vi "KRION6T_termo_main__.vi"() -> ()   [LabVIEW 2015]
doc: "Термометрия КРИОН-6Т"
uses:
  <vilib>/NI/Modbus Library/API/Master/Modbus Master.lvclass
  <vilib>/Utility/error.llb/DialogType.ctl
panel:
  in  "счетчик":u16
  out "Связь с блоком":bool
  in  "Tab Control":enum32{"ИЗМЕРЕНИЯ", "НАСТРОЙКИ"}(tab)
  out "Alarm":bool
  out "разница Т":dbl format="%.2f"
  in  "4_ch_visible":bool=TRUE
  in  "3_ch_visible":bool=TRUE
  out "R2":dbl format="%.2f"
  out "R1":dbl format="%.2f"
  in  "2_ch_visible":bool=TRUE
  in  "1_ch_visible":bool=TRUE
  out "Спаи":dbl format="%.2f"
  out "Cтр.":dbl format="%.2f"
  out "Пер.":dbl format="%.2f"
  out "Сол.":dbl format="%.2f"
  out "R3":dbl format="%.2f"
  out "R4":dbl format="%.2f"
  in  "Т min":dbl=4.0 min=-10.0 max=350.0 step=0.1
  in  "Т max":dbl=350.0 min=2.0 max=500.0 step=0.1
  in  "Autoscale":bool=TRUE
  out "сек.":string="0"
  out "часы":string="0"
  in  "Добавить время":dbl(ring)=300.0 items=["10 сек."=10.0, "1 мин."=60.0, "5 мин."=300.0, "20 мин."=1200.0]
  out "мин.":string="1"
  in  "xScale +":bool
  in  "xScale -":bool
  in  "Сохранение в файл":bool
  in  "Buf_size":u16=10 min=1 max=128
  in  "SPS":T1(ring)=enum."5 SPS"
  out "Путь к файлу с коэффициентами":path
  in  "Пароль":string
  in  "настр. коэфф.":bool caption="Disconn"
  in  "К спаи":T2 {"R0" format="%#_16g"; "k7" format="%#_16g"; "k6" format="%#_16g"; "k5" format="%#_16g"; "k4" format="%#_16g"; "k3" format="%#_16g"; "k2" format="%#_16g"; "k1" format="%#_16g"}
  in  "load_coeff.":bool caption="Disconn"
  in  "save_coeff.":bool caption="Disconn"
  in  "stop":bool
  in  "К стр.":T2 {"R0" format="%#_16g"; "k7" format="%#_16g"; "k6" format="%#_16g"; "k5" format="%#_16g"; "k4" format="%#_16g"; "k3" format="%#_16g"; "k2" format="%#_16g"; "k1" format="%#_16g"}
  in  "GraphLookB":bool
  in  "IP":string
  in  "Порт":u16
  in  "К пер.":T2 {"R0" format="%#_16g"; "k7" format="%#_16g"; "k6" format="%#_16g"; "k5" format="%#_16g"; "k4" format="%#_16g"; "k3" format="%#_16g"; "k2" format="%#_16g"; "k1" format="%#_16g"}
  in  "К сол.":T2 {"R0" format="%#_16g"; "k7" format="%#_16g"; "k6" format="%#_16g"; "k5" format="%#_16g"; "k4" format="%#_16g"; "k3" format="%#_16g"; "k2" format="%#_16g"; "k1" format="%#_16g"}
  out "Path":string
  in  "интервал сохр.":u16=10 min=1 max=3600 step=1
  out "Сутки":string
  in  "Запись в файл":bool
  out "File header exist?":bool caption="Disconn"
  in  "ADC_dyn_range":T3(ring)=enum."± 0.625 В"
  out "refnum out":refnum<file>
  out "Graphs T":dynamicdata(graph) caption="ИЗМЕРЕНИЯ ТЕМПЕРАТУРЫ, К"
  out "Связь":refnum<class "Modbus Master.lvclass">
  in  "Buf_size":u8=1 min=1 max=128
  in  "SPS":T1(ring)
  out "Расположение файла":path
  # "Т [K]"
  # "R [Ом]"
  # "сол./спаи dT ="
  # "Больше 40 К ?"
  # ":"
  # ":"
  # "Шкала Т"
  # "id 103"
  # "Скорость измерений"
  # "Размер буфера усредн."
  # "SPS = Samples Per Second"
  # "сек."
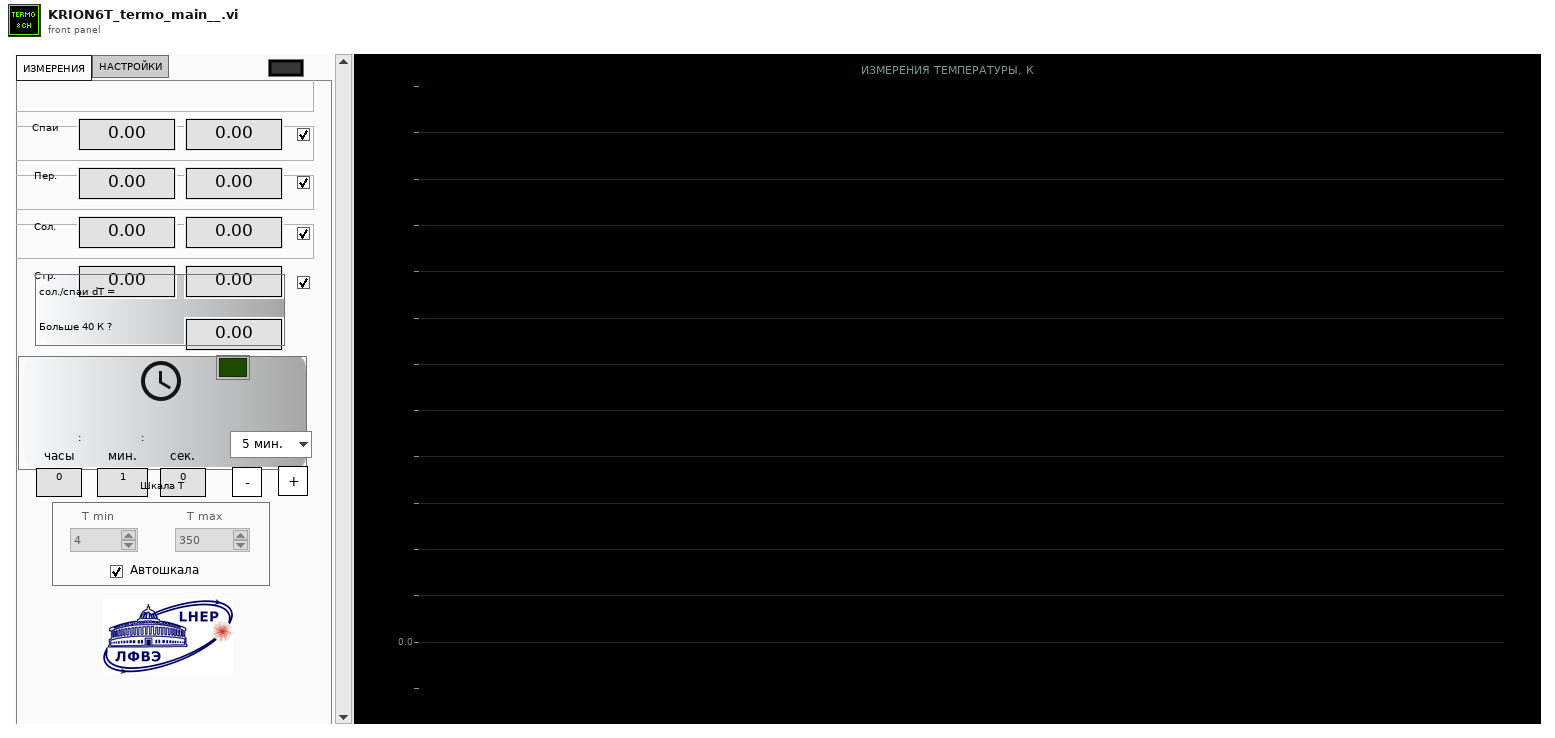
[diagram p1: front panel]
types:
  T1 = enum16{"2,5 SPS", "5 SPS", "10 SPS", "25 SPS", "50 SPS", "100 SPS", "500 SPS", "1 kSPS"}
  T2 = cluster{"k1":ext, "k2":ext, "k3":ext, "k4":ext, "k5":ext, "k6":ext, "k7":ext, "R0":ext}
  T3 = enum16{"± 5 В", "± 2.5 В", "± 1.25 В", "± 0.625 В", "± 312.5 мВ", "± 156.25 мВ", "± 78.125 мВ"}
  T4 = typedef "DialogType.ctl" = u16
  T5 = enum8{"Enabled", "Disabled", "Disabled and Grayed Out"}
  T6 = typedef "LVDateTimeRec.ctl" = cluster{"fractional second":dbl, "second":i32, "minute":i32, "hour":i32, "day of month":i32, "month":i32, "year":i32, "day of week":i32, "day of year":i32, "DST":i32}
  T7 = enum16{"open", "replace", "create", "open or create", "replace or create", "replace or create with confirmation"}
  T8 = cluster{"k1":ext, "k2":ext, "k3":ext, "k4":ext, "k5":ext, "k6":ext, "k7":ext, "R":ext}
  T9 = cluster{"Cтр.":dbl, "Спаи":dbl, "Пер.":dbl, "Сол.":dbl}
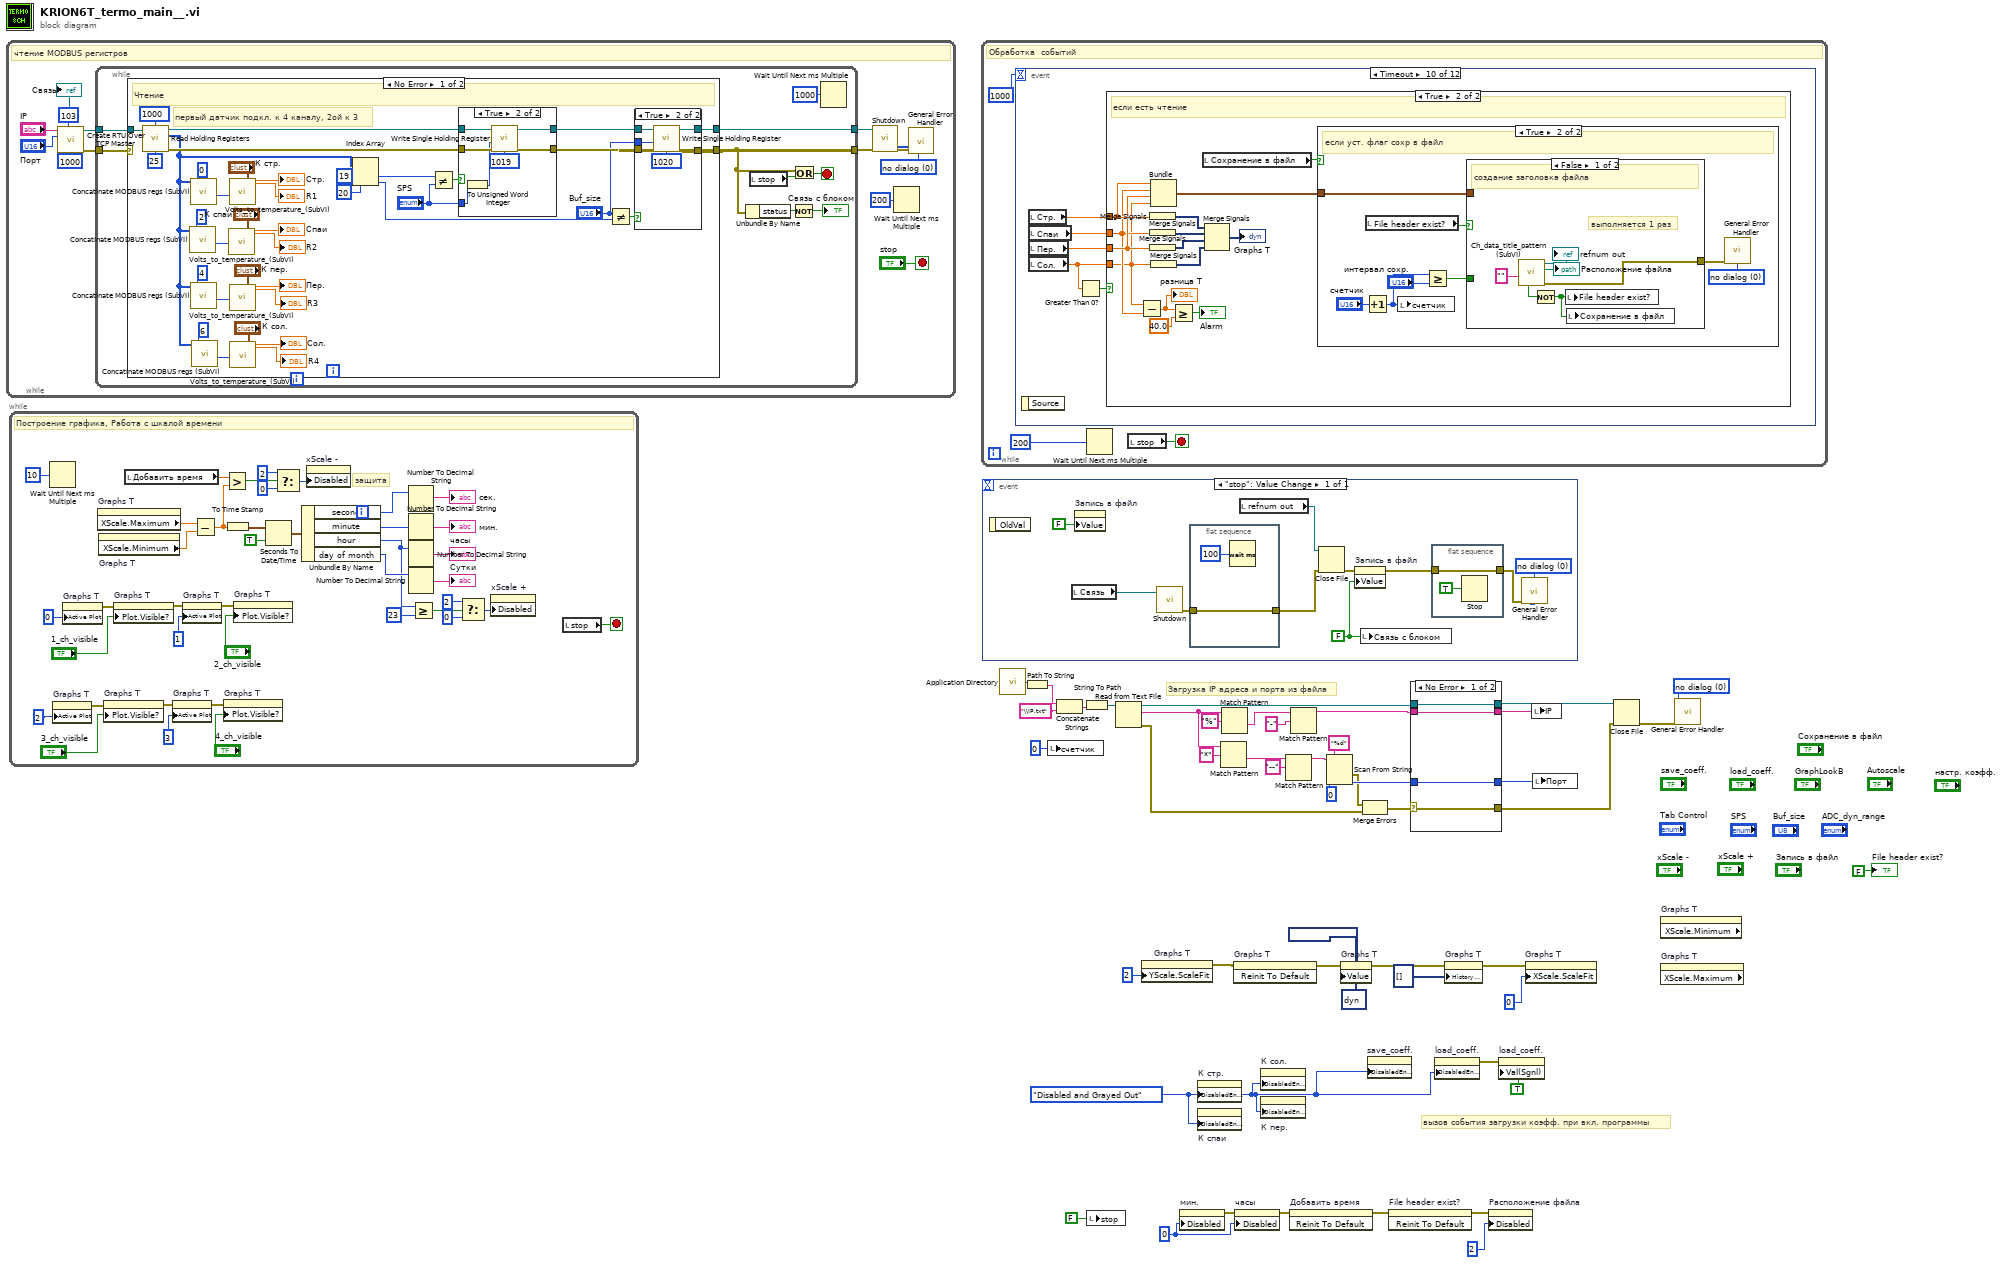
[diagram p0: block diagram]
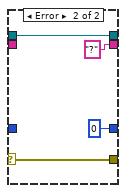
[diagram p2: hidden frame]
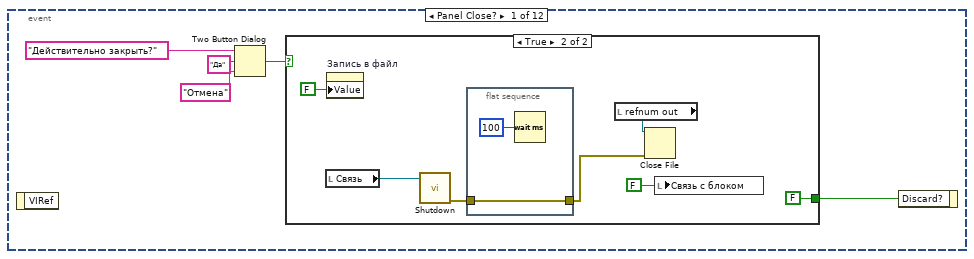
[diagram p3: hidden frame]
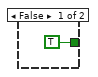
[diagram p4: hidden frame]
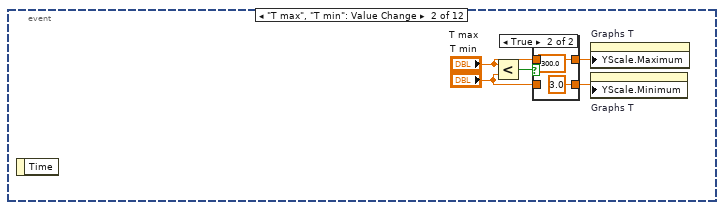
[diagram p5: hidden frame]
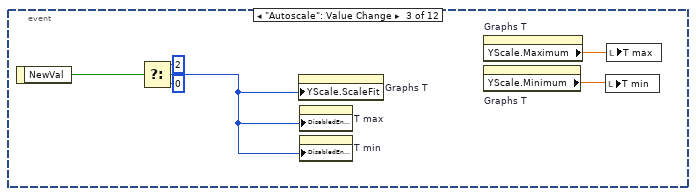
[diagram p7: hidden frame]
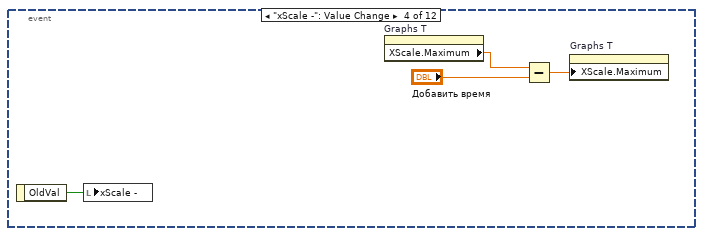
[diagram p8: hidden frame]
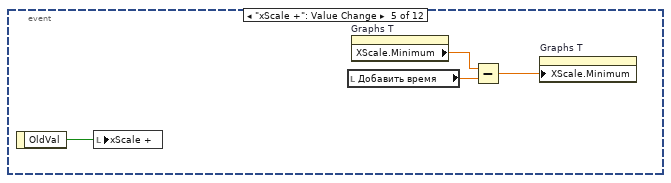
[diagram p9: hidden frame]
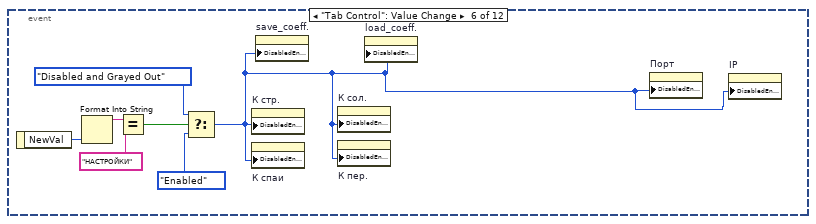
[diagram p10: hidden frame]
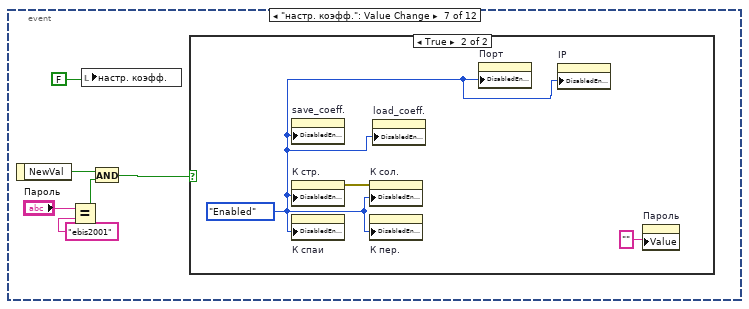
[diagram p11: hidden frame]
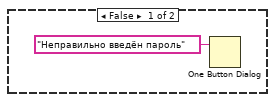
[diagram p12: hidden frame]
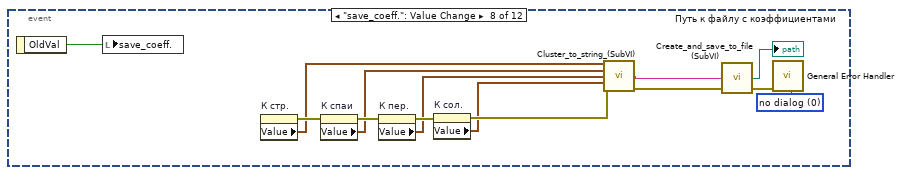
[diagram p13: hidden frame]
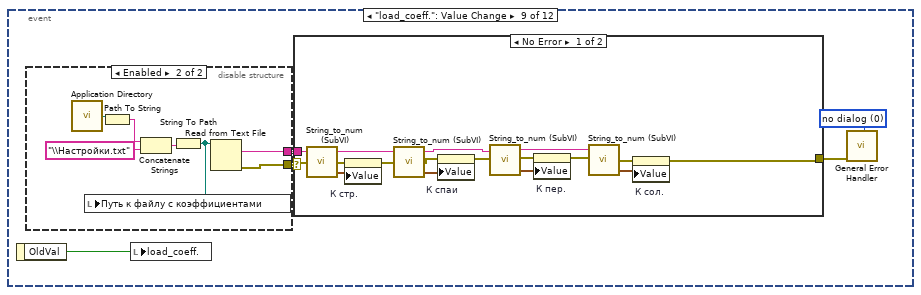
[diagram p14: hidden frame]
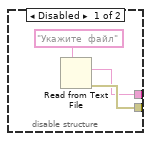
[diagram p15: hidden frame]
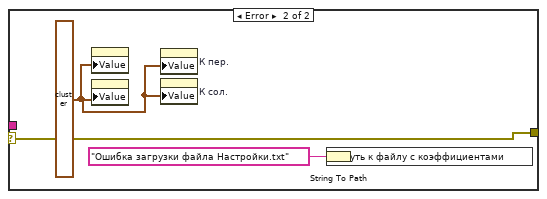
[diagram p16: hidden frame]
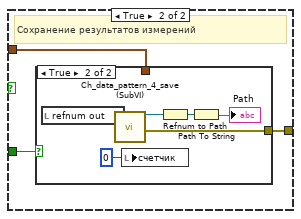
[diagram p19: hidden frame]
diagram:
  w12 = T4 0 items=["no dialog", "OK message", "continue or stop message", "OK message + warnings", "continue/stop + warnings"] ("type of dialog (OK msg:1)")
  w2 = T5."Disabled and Grayed Out" ("Disabled")
  w46 = u8 0 ("Disabled")
  # "Загрузка IP адреса и порта из файла"
  # "вызов события загрузки коэфф. при вкл. программы"
  n1 = while {
    stop <- "stop" stop-if-true
    w48 = T4 0 items=["no dialog", "OK message", "continue or stop message", "OK message + warnings", "continue/stop + warnings"] ("type of dialog (OK msg:1)")
    # "чтение MODBUS регистров"
    n2 = call "Create RTU Over TCP Master.vi"("unit ID"=u8 103 ("ID"), "connect timeout ms"=1000, "port (502)"="Порт", "address"="IP") -> ("error out"=w52:errorcluster, "TCP master instance"=w53:refnum<class "Modbus Master.lvclass">)  [unwired: 6 in]
    "Связь" <- w53
    n3 = while {
      tunnel: w53 -> [w68]
      tunnel: w52 -> [w67]
      tunnel: [w61] -> w51
      tunnel: [w66] -> w50
      stop <- w64 stop-if-true
      n4 = case shown="No Error" w67 {
        selector: w67 -> [_ w126]
        tunnel: w68 -> [w104 w127]
        tunnel: [w80 w126] -> w61
        tunnel: [w81 w127] -> w66
        frame No Error {
          # "первый датчик подкл. к 4 каналу, 2ой к 3"
          # "Чтение"
          n5 = call-dynamic "Read Holding Registers.vi"("number of inputs"=u16 25, "starting address"=u16 1000, "Modbus master in"=w104) -> ("error out"=w78:errorcluster, "register values"=w77:u16[], "Modbus master out"=w79:refnum<class "Modbus Master.lvclass">)  [unwired: 6 in]
          n6 = call "Concatinate MODBUS regs (SubVI).vi"("LSB reg num"=u16 2, "registers array in"=w77) -> ("register data"=w99:i32)  [unwired: 8 in, 1 out]
          n7 = call "Concatinate MODBUS regs (SubVI).vi"("LSB reg num"=u16 0, "registers array in"=w77) -> ("register data"=w101:i32)  [unwired: 8 in, 1 out]
          n8 = call "Concatinate MODBUS regs (SubVI).vi"("LSB reg num"=u16 4, "registers array in"=w77) -> ("register data"=w90:i32)  [unwired: 8 in, 1 out]
          n9 = call "Concatinate MODBUS regs (SubVI).vi"("LSB reg num"=u16 6, "registers array in"=w77) -> ("register data"=w87:i32)  [unwired: 8 in, 1 out]
          n10 = call "Volts_to_temperature_(SubVI).vi"("Resistance"=w99, "koeff. cluster"="К спаи") -> ("T solvation"=→"Спаи":dbl, "meas_voltage"=→"R2":dbl)  [unwired: 21 in, 3 out]
          n11 = call "Volts_to_temperature_(SubVI).vi"("Resistance"=w101, "koeff. cluster"="К стр.") -> ("T solvation"=→"Cтр.":dbl, "meas_voltage"=→"R1":dbl)  [unwired: 21 in, 3 out]
          n12 = call "Volts_to_temperature_(SubVI).vi"("Resistance"=w90, "koeff. cluster"="К пер.") -> ("T solvation"=→"Пер.":dbl, "meas_voltage"=→"R3":dbl)  [unwired: 21 in, 3 out]
          n13 = call "Volts_to_temperature_(SubVI).vi"("Resistance"=w87, "koeff. cluster"="К сол.") -> ("T solvation"=→"Сол.":dbl, "meas_voltage"=→"R4":dbl)  [unwired: 21 in, 3 out]
          n14 = Index Array(array=w77, index #1=19 ("index"), index #2=20 ("index")) -> (element #1=w76:u16, element #2=w70:u16)
          n15 = Not Equal?(x=w76, y="SPS") -> (x != y?=w75:bool)
          n16 = case shown="True" w75 {
            tunnel: w79 -> [w116 w123]
            tunnel: w78 -> [w115 w122]
            tunnel: [w116 w120] -> w83
            tunnel: [w115 w119] -> w82
            tunnel: "SPS" -> [_ w118]
            frame False {
            }
            frame True {
              n17 = To Unsigned Word Integer(number=w118) -> (unsigned 16bit integer=w117:u16)
              n18 = call-dynamic "Write Single Holding Register.vi"("error in"=w122, "register to write"=w117, "address"=u16 1019 ("starting address"), "Modbus master in"=w123) -> ("error out"=w119:errorcluster, "Modbus master out"=w120:refnum<class "Modbus Master.lvclass">)  [unwired: 6 in]
            }
          }
          n19 = Not Equal?(x="Buf_size", y=w70) -> (x != y?=w71:bool)
          n20 = case shown="True" w71 {
            tunnel: w83 -> [w108 w114]
            tunnel: w82 -> [w107 w113]
            tunnel: [w108 w111] -> w81
            tunnel: [w107 w110] -> w80
            tunnel: "Buf_size" -> [_ w109]
            frame False {
            }
            frame True {
              n21 = call-dynamic "Write Single Holding Register.vi"("error in"=w113, "register to write"=w109, "address"=u16 1020 ("starting address"), "Modbus master in"=w114) -> ("error out"=w110:errorcluster, "Modbus master out"=w111:refnum<class "Modbus Master.lvclass">)  [unwired: 6 in]
            }
          }
        }
        frame Error {
          w124 = -1.0 ("R1")
          w125 = -1.0 ("R1")
          n22 = local write "R1"(w125) -> ()
          n23 = local write "R2"(w125) -> ()
          n24 = local write "R3"(w125) -> ()
          n25 = local write "R4"(w125) -> ()
          n26 = local write "Cтр."(w124) -> ()
          n27 = local write "Спаи"(w124) -> ()
          n28 = local write "Пер."(w124) -> ()
          n29 = local write "Сол."(w124) -> ()
        }
      }
      n30 = Unbundle By Name(w61) -> ("status"=w63:bool)
      n31 = local read "stop"() -> (w65:bool)
      n32 = Not(x=w63) -> (.not. x?=→"Связь с блоком":bool)
      n33 = Or(x=w61, y=w65) -> (x .or. y?=w64:bool)
      n34 = Wait Until Next ms Multiple(millisecond multiple=u32 1000) -> ()  [unwired: 1 out]
    }
    n35 = call-dynamic "Shutdown.vi"("error in"=w51, "Modbus master in"=w50) -> ("error out"=w49:errorcluster)  [unwired: 9 in]
    n36 = Wait Until Next ms Multiple(millisecond multiple=u32 200) -> ()  [unwired: 1 out]
    n37 = call <vilib>:"General Error Handler.vi"("type of dialog (OK msg:1)"=w48, "error in (no error)"=w49) -> ()  [unwired: 1 in, 13 out]
  }
  n38 = while {
    stop <- w167 stop-if-true
    # "защита"
    # "Построение графика, Работа с шкалой времени"
    n39 = Wait Until Next ms Multiple(millisecond multiple=u32 10) -> ()  [unwired: 1 out]
    n40 = property on="Graphs T" class="WFChart (strict)"("Active Plot"=u32 2) -> (error out=w134:errorcluster)  [unwired: 2 in, 1 out]
    n41 = property on="Graphs T" class="WFChart (strict)"("Active Plot"=u32 0) -> (error out=w135:errorcluster)  [unwired: 2 in, 1 out]
    n42 = property on="Graphs T" class="WFChart (strict)"() -> ("XScale.Maximum"=w143:dbl)  [unwired: 2 in, 2 out]
    n43 = property on="Graphs T" class="WFChart (strict)"() -> ("XScale.Minimum"=w142:dbl)  [unwired: 2 in, 2 out]
    n44 = property on="Graphs T" class="WFChart (strict)"(error in=w134, "Plot.Visible?"="3_ch_visible") -> (error out=w129:errorcluster)  [unwired: 1 in, 1 out]
    n45 = property on="Graphs T" class="WFChart (strict)"(error in=w135, "Plot.Visible?"="1_ch_visible") -> (error out=w140:errorcluster)  [unwired: 1 in, 1 out]
    n46 = local read "Добавить время"() -> (w166:dbl)
    n47 = property on="Graphs T" class="WFChart (strict)"(error in=w129, "Active Plot"=u32 3) -> (error out=w131:errorcluster)  [unwired: 1 in, 1 out]
    n48 = property on="Graphs T" class="WFChart (strict)"(error in=w140, "Active Plot"=u32 1) -> (error out=w138:errorcluster)  [unwired: 1 in, 1 out]
    n49 = Subtract(x=w143, y=w142) -> (x-y=w156:dbl)
    n50 = property on="Graphs T" class="WFChart (strict)"(error in=w131, "Plot.Visible?"="4_ch_visible") -> ()  [unwired: 1 in, 2 out]
    n51 = Greater?(x=w166, y=w156) -> (0:w149:bool)
    n52 = To Time Stamp(1:w156) -> (0:w164:timestamp)
    n53 = property on="Graphs T" class="WFChart (strict)"(error in=w138, "Plot.Visible?"="2_ch_visible") -> ()  [unwired: 1 in, 2 out]
    n54 = Seconds To Date/Time(time stamp (now)=w164, to UTC (F)=TRUE) -> (date time rec=w163:T6)
    n55 = Select(t=u8 2 ("Disabled"), s=w149, f=u8 0 ("Disabled")) -> (s? t:f=w152:u8)
    n56 = Unbundle By Name(w163) -> ("second"=w162:i32, "minute"=w161:i32, "hour"=w154:i32, "day of month"=w160:i32)
    n57 = property on="xScale -" class="Bool (strict)"("Disabled"=w152) -> ()  [unwired: 2 in, 2 out]
    n58 = Number To Decimal String(number=w162) -> (decimal integer string=→"сек.":string)  [unwired: 1 out]
    n59 = Number To Decimal String(number=w161) -> (decimal integer string=→"мин.":string)  [unwired: 1 out]
    n60 = Number To Decimal String(number=w154) -> (decimal integer string=→"часы":string)  [unwired: 1 out]
    n61 = Number To Decimal String(number=w160) -> (decimal integer string=→"Сутки":string)  [unwired: 1 out]
    n62 = Greater Or Equal?(x=w154, y=23) -> (x >= y?=w145:bool)
    n63 = Select(t=u8 2 ("Disabled"), s=w145, f=u8 0 ("Disabled")) -> (s? t:f=w148:u8)
    n64 = property on="xScale +" class="Bool (strict)"("Disabled"=w148) -> ()  [unwired: 2 in, 2 out]
    n65 = local read "stop"() -> (w167:bool)
  }
  n66 = while {
    stop <- w169 stop-if-true
    # "Обработка  событий"
    n67 = event shown="[9] Timeout" {
      selector: _ -> [_ _ _ _ _ _ _ _ _ _ _ _]
      dyn-events: _ -> [_ _ _ _ _ _ _ _ _ _ _ _]
      timeout: 1000 -> [_ _ _ _ _ _ _ _ _ _ _ _]
      event Panel Close? {
        n68 = event-data() -> ()  [unwired: 2 out]
        n69 = Two Button Dialog(message="Действительно закрыть?", 1:"Отмена" ("T button name (\"OK\")"), 2:"Да" ("T button name (\"OK\")")) -> (T button?=w175:bool)
        n70 = case shown="True" w175 {
          tunnel: [TRUE ("Discard?") FALSE ("Discard?")] -> w171
          frame False {
          }
          frame True {
            n71 = local read "Связь"() -> (w180:refnum<class "Modbus Master.lvclass">)
            n72 = property on="Запись в файл" class="Bool (strict)"("Value"=FALSE ("Запись в файл")) -> ()  [unwired: 2 in, 2 out]
            n73 = call-dynamic "Shutdown.vi"("Modbus master in"=w180) -> ("error out"=w179:errorcluster)  [unwired: 10 in]
            n74 = flat-sequence {
              tunnel: w179 -> [w184]
              tunnel: [w184] -> w178
              frame #0 {
                n75 = Wait (ms)(milliseconds to wait=u32 100) -> ()  [unwired: 1 out]
              }
            }
            n76 = local read "refnum out"() -> (w182:refnum<file>)
            n77 = Close File(refnum=w182, error in=w178) -> ()  [unwired: 2 out]
            n78 = local write "Связь с блоком"(FALSE ("Связь с блоком 4")) -> ()
          }
        }
        n79 = event-data("Discard?"=w171) -> ()  [unwired: 1 in, 1 out]
      }
      event "Т max", "Т min": Value Change {
        n80 = event-data() -> ()  [unwired: 2 out]
        n81 = Less?(x="Т max", y="Т min") -> (x < y?=w190:bool)
        n82 = case shown="True" w190 {
          tunnel: [w191 300.0 ("x+1")] -> w188
          tunnel: [w192 3.0 ("x+1")] -> w189
          tunnel: "Т max" -> [w191 _]
          tunnel: "Т min" -> [w192 _]
          frame False {
          }
          frame True {
          }
        }
        n83 = property on="Graphs T" class="WFChart (strict)"("YScale.Maximum"=w188) -> ()  [unwired: 2 in, 2 out]
        n84 = property on="Graphs T" class="WFChart (strict)"("YScale.Minimum"=w189) -> ()  [unwired: 2 in, 2 out]
      }
      event "Autoscale": Value Change {
        n85 = event-data() -> ("NewVal"=w195:bool)  [unwired: 1 out]
        n86 = Select(t=u8 2 ("Y Scale.Scale Fit"), s=w195, f=u8 0 ("Y Scale.Scale Fit")) -> (s? t:f=w198:u8)
        n87 = property on="Graphs T" class="WFChart (strict)"("YScale.ScaleFit"=w198) -> ()  [unwired: 2 in, 2 out]
        n88 = property on="Т max" class="DigNum (strict)"("DisabledEnum"=w198) -> ()  [unwired: 2 in, 2 out]
        n89 = property on="Т min" class="DigNum (strict)"("DisabledEnum"=w198) -> ()  [unwired: 2 in, 2 out]
        n90 = property on="Graphs T" class="WFChart (strict)"() -> ("YScale.Maximum"=w200:dbl)  [unwired: 2 in, 2 out]
        n91 = property on="Graphs T" class="WFChart (strict)"() -> ("YScale.Minimum"=w199:dbl)  [unwired: 2 in, 2 out]
        n92 = local write "Т min"(w199) -> ()
        n93 = local write "Т max"(w200) -> ()
      }
      event "xScale -": Value Change {
        n94 = event-data() -> ("OldVal"=w204:bool)  [unwired: 1 out]
        n95 = local write "xScale -"(w204) -> ()
        n96 = property on="Graphs T" class="WFChart (strict)"() -> ("XScale.Maximum"=w202:dbl)  [unwired: 2 in, 2 out]
        n97 = Subtract(x=w202, y="Добавить время") -> (x-y=w201:dbl)
        n98 = property on="Graphs T" class="WFChart (strict)"("XScale.Maximum"=w201) -> ()  [unwired: 2 in, 2 out]
      }
      event "xScale +": Value Change {
        n99 = event-data() -> ("OldVal"=w208:bool)  [unwired: 1 out]
        n100 = local write "xScale +"(w208) -> ()
        n101 = local read "Добавить время"() -> (w207:dbl)
        n102 = property on="Graphs T" class="WFChart (strict)"() -> ("XScale.Minimum"=w206:dbl)  [unwired: 2 in, 2 out]
        n103 = Subtract(x=w206, y=w207) -> (x-y=w205:dbl)
        n104 = property on="Graphs T" class="WFChart (strict)"("XScale.Minimum"=w205) -> ()  [unwired: 2 in, 2 out]
      }
      event "Tab Control": Value Change {
        n105 = event-data() -> ("NewVal"=w215:enum32{"ИЗМЕРЕНИЯ", "НАСТРОЙКИ"})  [unwired: 1 out]
        n106 = Format Into String(w215) -> (resulting string=w214:string)  [unwired: 3 in, 1 out]
        n107 = Equal?(x=w214, y="НАСТРОЙКИ") -> (x = y?=w212:bool)
        n108 = Select(t=T5."Disabled and Grayed Out" ("Disabled"), s=w212, f=T5."Enabled" ("Disabled")) -> (s? t:f=w209:T5)
        n109 = property on="К стр." class="Clust (strict)"("DisabledEnum"=w209) -> ()  [unwired: 2 in, 2 out]
        n110 = property on="К спаи" class="Clust (strict)"("DisabledEnum"=w209) -> ()  [unwired: 2 in, 2 out]
        n111 = property on="save_coeff." class="Bool (strict)"("DisabledEnum"=w209) -> ()  [unwired: 2 in, 2 out]
        n112 = property on="К сол." class="Clust (strict)"("DisabledEnum"=w209) -> ()  [unwired: 2 in, 2 out]
        n113 = property on="К пер." class="Clust (strict)"("DisabledEnum"=w209) -> ()  [unwired: 2 in, 2 out]
        n114 = property on="load_coeff." class="Bool (strict)"("DisabledEnum"=w209) -> ()  [unwired: 2 in, 2 out]
        n115 = property on="Порт" class="DigNum (strict)"("DisabledEnum"=w209) -> ()  [unwired: 2 in, 2 out]
        n116 = property on="IP" class="Str"("DisabledEnum"=w209) -> ()  [unwired: 2 in, 2 out]
      }
      event "настр. коэфф.": Value Change {
        n117 = event-data() -> ("NewVal"=w221:bool)  [unwired: 1 out]
        n118 = Equal?(x="Пароль", y="ebis2001") -> (x = y?=w218:bool)
        n119 = local write "настр. коэфф."(FALSE ("насстр. коэфф.")) -> ()
        n120 = And(x=w221, y=w218) -> (x .and. y?=w217:bool)
        n121 = case shown="True" w217 {
          frame False {
            n122 = One Button Dialog(message="Неправильно введён пароль") -> ()  [unwired: 1 in, 1 out]
          }
          frame True {
            w223 = T5."Enabled" ("Disabled")
            n123 = property on="save_coeff." class="Bool (strict)"("DisabledEnum"=w223) -> ()  [unwired: 2 in, 2 out]
            n124 = property on="К стр." class="Clust (strict)"("DisabledEnum"=w223) -> (error out=w224:errorcluster)  [unwired: 2 in, 1 out]
            n125 = property on="К спаи" class="Clust (strict)"("DisabledEnum"=w223) -> ()  [unwired: 2 in, 2 out]
            n126 = property on="К сол." class="Clust (strict)"(error in=w224, "DisabledEnum"=w223) -> ()  [unwired: 1 in, 2 out]
            n127 = property on="К пер." class="Clust (strict)"("DisabledEnum"=w223) -> ()  [unwired: 2 in, 2 out]
            n128 = property on="load_coeff." class="Bool (strict)"("DisabledEnum"=w223) -> ()  [unwired: 2 in, 2 out]
            n129 = property on="Порт" class="DigNum (strict)"("DisabledEnum"=w223) -> ()  [unwired: 2 in, 2 out]
            n130 = property on="IP" class="Str"("DisabledEnum"=w223) -> ()  [unwired: 2 in, 2 out]
            n131 = property on="Пароль" class="Str"("Value"="" ("Пароль")) -> ()  [unwired: 2 in, 2 out]
          }
        }
      }
      event "save_coeff.": Value Change {
        w234 = T4 0 items=["no dialog", "OK message", "continue or stop message", "OK message + warnings", "continue/stop + warnings"] ("type of dialog (OK msg:1)")
        n132 = event-data() -> ("OldVal"=w239:bool)  [unwired: 1 out]
        n133 = local write "save_coeff."(w239) -> ()
        n134 = property on="К стр." class="Clust (strict)"() -> (error out=w238:errorcluster, "Value"=w237:T2)  [unwired: 2 in, 1 out]
        n135 = property on="К спаи" class="Clust (strict)"(error in=w238) -> (error out=w231:errorcluster, "Value"=w228:T2)  [unwired: 1 in, 1 out]
        n136 = property on="К пер." class="Clust (strict)"(error in=w231) -> (error out=w230:errorcluster, "Value"=w227:T2)  [unwired: 1 in, 1 out]
        n137 = property on="К сол." class="Clust (strict)"(error in=w230) -> (error out=w229:errorcluster, "Value"=w226:T2)  [unwired: 1 in, 1 out]
        n138 = call "Cluster_to_string_(SubVI).vi"("input cluster 1"=w237, "input cluster 2"=w228, "input cluster 3"=w227, "input cluster 4"=w226, "error in"=w229) -> ("string of coefficients"=w232:string, "error out"=w236:errorcluster)  [unwired: 9 in]
        n139 = call "Create_and_save_to_file (SubVI).vi"("input string"=w232, "error in"=w236) -> ("Текущее расположение файла"=→"Путь к файлу с коэффициентами":path, "error out"=w235:errorcluster)  [unwired: 4 in]
        n140 = call <vilib>:"General Error Handler.vi"("type of dialog (OK msg:1)"=w234, "error in (no error)"=w235) -> ()  [unwired: 9 in, 5 out]
      }
      event "load_coeff.": Value Change {
        w242 = T4 0 items=["no dialog", "OK message", "continue or stop message", "OK message + warnings", "continue/stop + warnings"] ("type of dialog (OK msg:1)")
        n141 = event-data() -> ("OldVal"=w244:bool)  [unwired: 1 out]
        n142 = disable-structure shown="Enabled" {
          disable-tunnel: [w247 w250] -> w241
          disable-tunnel: [w246 w251] -> w243
          frame Disabled {
            n143 = Read from Text File(prompt (Open existing file)="Укажите  файл") -> (text=w246:string, cancelled=w248:bool, error out=w247:errorcluster)  [unwired: 3 in, 1 out]
          }
          frame Enabled {
            n144 = call <vilib>:"Application Directory.vi"() -> ("Application Directory"=w255:path)
            n145 = Path To String(path=w255) -> (string=w254:string)
            n146 = Concatenate Strings(w254, "\\Настройки.txt" ("prompt (Open existing file)")) -> (w253:string)
            n147 = String To Path(string=w253) -> (path=w249:path)
            n148 = local write "Путь к файлу с коэффициентами"(w249) -> ()
            n149 = Read from Text File(file (use dialog)=w249) -> (text=w251:string, error out=w250:errorcluster)  [unwired: 3 in, 2 out]
          }
        }
        n150 = local write "load_coeff."(w244) -> ()
        n151 = case shown="No Error" w241 {
          selector: w241 -> [w265 w274]
          tunnel: w243 -> [w272 _]
          tunnel: [w256 w274] -> w240
          frame No Error {
            n152 = call "String_to_num (SubVI).vi"("String in"=w272, "error in"=w265) -> ("Rest of string OUT"=w269:string, "error out"=w270:errorcluster, "output cluster \nof coefficients"=w271:T8)  [unwired: 5 in]
            n153 = property on="К стр." class="Clust (strict)"(error in=w270, "Value"=w271) -> (error out=w268:errorcluster)  [unwired: 1 in, 1 out]
            n154 = call "String_to_num (SubVI).vi"("String in"=w269, "error in"=w268) -> ("Rest of string OUT"=w261:string, "error out"=w267:errorcluster, "output cluster \nof coefficients"=w266:T8)  [unwired: 5 in]
            n155 = property on="К спаи" class="Clust (strict)"(error in=w267, "Value"=w266) -> (error out=w264:errorcluster)  [unwired: 1 in, 1 out]
            n156 = call "String_to_num (SubVI).vi"("String in"=w261, "error in"=w264) -> ("Rest of string OUT"=w260:string, "error out"=w262:errorcluster, "output cluster \nof coefficients"=w263:T8)  [unwired: 5 in]
            n157 = property on="К пер." class="Clust (strict)"(error in=w262, "Value"=w263) -> (error out=w259:errorcluster)  [unwired: 1 in, 1 out]
            n158 = call "String_to_num (SubVI).vi"("String in"=w260, "error in"=w259) -> ("error out"=w258:errorcluster, "output cluster \nof coefficients"=w257:T8)  [unwired: 5 in, 1 out]
            n159 = property on="К сол." class="Clust (strict)"(error in=w258, "Value"=w257) -> (error out=w256:errorcluster)  [unwired: 1 in, 1 out]
          }
          frame Error {
            w273 = T2 {"k1"=0.0, "k2"=0.0, "k3"=0.0, "k4"=0.0, "k5"=0.0, "k6"=0.0, "k7"=0.0, "R0"=0.0} ("Coeff_cl_ch1")
            n160 = property on="К стр." class="Clust (strict)"("Value"=w273) -> ()  [unwired: 2 in, 2 out]
            n161 = property on="К спаи" class="Clust (strict)"("Value"=w273) -> ()  [unwired: 2 in, 2 out]
            n162 = property on="К пер." class="Clust (strict)"("Value"=w273) -> ()  [unwired: 2 in, 2 out]
            n163 = property on="К сол." class="Clust (strict)"("Value"=w273) -> ()  [unwired: 2 in, 2 out]
            n164 = String To Path(string="Ошибка загрузки файла Настройки.txt") -> (path=w276:path)
            n165 = local write "Путь к файлу с коэффициентами"(w276) -> ()
          }
        }
        n166 = call <vilib>:"General Error Handler.vi"("type of dialog (OK msg:1)"=w242, "error in (no error)"=w240) -> ()  [unwired: 9 in, 5 out]
      }
      event Timeout {
        n167 = event-data() -> ()  [unwired: 2 out]
        n168 = local read "Cтр."() -> (w281:dbl)
        n169 = local read "Спаи"() -> (w279:dbl)
        n170 = local read "Пер."() -> (w280:dbl)
        n171 = local read "Сол."() -> (w278:dbl)
        n172 = Greater Than 0?(x=w278) -> (x > 0?=w277:bool)
        n173 = case shown="True" w277 {
          tunnel: w281 -> [_ w290]
          tunnel: w280 -> [_ w289]
          tunnel: w279 -> [_ w287]
          tunnel: w278 -> [_ w283]
          frame False {
          }
          frame True {
            # "если есть чтение"
            n174 = Subtract(x=w283, y=w287) -> (x-y=w285:dbl)
            "разница Т" <- w285
            n175 = Merge Signals(w290) -> (w295:dynamicdata)
            n176 = Merge Signals(w287) -> (w294:dynamicdata)
            n177 = Merge Signals(w289) -> (w293:dynamicdata)
            n178 = Bundle("Cтр."=w290, "Спаи"=w287, "Пер."=w289, "Сол."=w283) -> (w288:T9)  [unwired: 1 in]
            n179 = Merge Signals(w283) -> (w292:dynamicdata)
            n180 = Greater Or Equal?(x=w285, y=40.0) -> (x >= y?=→"Alarm":bool)
            n181 = local read "Сохранение в файл"() -> (w282:bool)
            n182 = Merge Signals(w295, w294, w293, w292) -> (→"Graphs T":dynamicdata)
            n183 = case shown="True" w282 {
              tunnel: w288 -> [_ w303]
              frame False {
              }
              frame True {
                w302 = T4 0 items=["no dialog", "OK message", "continue or stop message", "OK message + warnings", "continue/stop + warnings"] ("type of dialog (OK msg:1)")
                # "если уст. флаг сохр в файл"
                n184 = Increment(x="счетчик") -> (x+1=w299:u16)
                n185 = local read "File header exist?"() -> (w297:bool)
                n186 = local write "счетчик"(w299) -> ()
                n187 = Greater Or Equal?(x=w299, y="интервал сохр.") -> (x >= y?=w298:bool)
                n188 = case shown="False" w297 {
                  tunnel: w303 -> [_ w312]
                  tunnel: [w306 w311] -> w301
                  tunnel: w298 -> [_ w310]
                  frame False {
                    # "выполняется 1 раз"
                    # "создание заголовка файла"
                    n189 = call "Ch_data_title_pattern (SubVI).vi"("Единица измерений"="") -> ("error out"=w306:errorcluster, "Path"=→"Расположение файла":path, "Byte Stream File out"=→"refnum out":refnum<file>, "cancelled"=w305:bool)  [unwired: 7 in]
                    n190 = Not(x=w305) -> (.not. x?=w304:bool)
                    n191 = local write "File header exist?"(w304) -> ()
                    n192 = local write "Сохранение в файл"(w304) -> ()
                  }
                  frame True {
                    # "Сохранение результатов измерений"
                    n193 = case shown="True" w310 {
                      tunnel: w312 -> [_ _]
                      tunnel: [_ w313] -> w311
                      frame False {
                      }
                      frame True {
                        n194 = local read "refnum out"() -> (w317:refnum<file>)
                        n195 = call "Ch_data_pattern_4_save (SubVI).vi"() -> ("error out"=w313:errorcluster)  [unwired: 27 in]
                        n196 = local write "счетчик"(u8 0 ("счетчик")) -> ()
                        n197 = Refnum to Path(1:w317) -> (0:w316:path)
                        n198 = Path To String(path=w316) -> (string=→"Path":string)
                      }
                    }
                  }
                }
                n199 = call <vilib>:"General Error Handler.vi"("type of dialog (OK msg:1)"=w302, "error in (no error)"=w301) -> ()  [unwired: 1 in, 13 out]
              }
            }
          }
        }
      }
      event "Сохранение в файл": Value Change {
        n200 = event-data() -> ("NewVal"=w318:bool)  [unwired: 1 out]
        n201 = case shown="False" w318 {
          frame False {
            n202 = local write "File header exist?"(FALSE ("File header exist?")) -> ()
          }
          frame True {
          }
        }
      }
      event "IP", "Порт": Value Change {
        w323 = T4 0 items=["no dialog", "OK message", "continue or stop message", "OK message + warnings", "continue/stop + warnings"] ("type of dialog (OK msg:1)")
        n203 = event-data() -> ()  [unwired: 2 out]
        n204 = call <vilib>:"Application Directory.vi"() -> ("Application Directory"=w341:path)
        n205 = local read "IP"() -> (w337:string)
        n206 = local read "Порт"() -> (w336:u16)
        n207 = Path To String(path=w341) -> (string=w340:string)
        n208 = Concatenate Strings(w340, "\\IP.txt" ("prompt (Open existing file)")) -> (w339:string)
        n209 = Number To Decimal String(number=w336) -> (decimal integer string=w332:string)  [unwired: 1 in]
        n210 = String To Path(string=w339) -> (path=w324:path)
        n211 = Open/Create/Replace File(file path (use dialog)=w324, operation (0:open)=T7."replace or create") -> (refnum out=w327:refnum<file>, error out=w326:errorcluster)  [unwired: 1 in, 4 out]
        n212 = Concatenate Strings("%" ("string"), w337, "-" ("string")) -> (w333:string)
        n213 = Concatenate Strings("*" ("string"), w332, "--" ("string")) -> (w334:string)
        n214 = Concatenate Strings(w333, w334) -> (w335:string)
        n215 = Write to Text File(file (use dialog)=w327, text=w335, error in=w326) -> (refnum out=w329:refnum<file>, error out=w328:errorcluster)  [unwired: 2 out]
        n216 = Close File(refnum=w329, error in=w328) -> (error out=w322:errorcluster)  [unwired: 1 out]
        n217 = call <vilib>:"General Error Handler.vi"("type of dialog (OK msg:1)"=w323, "error in (no error)"=w322) -> ()  [unwired: 1 in, 13 out]
      }
    }
    n218 = Wait Until Next ms Multiple(millisecond multiple=u32 200) -> ()  [unwired: 1 out]
    n219 = local read "stop"() -> (w169:bool)
  }
  n220 = event shown="[0] \"stop\": Value Change" {
    selector: _ -> [_]
    dyn-events: _ -> [_]
    timeout: _ -> [_]
    event "stop": Value Change {
      w345 = T4 0 items=["no dialog", "OK message", "continue or stop message", "OK message + warnings", "continue/stop + warnings"] ("type of dialog (OK msg:1)")
      w342 = FALSE ("Запись в файл")
      n221 = event-data() -> ()  [unwired: 1 in, 1 out]
      n222 = local read "Связь"() -> (w347:refnum<class "Modbus Master.lvclass">)
      n223 = property on="Запись в файл" class="Bool (strict)"("Value"=FALSE ("Запись в файл")) -> ()  [unwired: 2 in, 2 out]
      n224 = call-dynamic "Shutdown.vi"("Modbus master in"=w347) -> ("error out"=w346:errorcluster)  [unwired: 10 in]
      n225 = flat-sequence {
        tunnel: w346 -> [w354]
        tunnel: [w354] -> w343
        frame #0 {
          n226 = Wait (ms)(milliseconds to wait=u32 100) -> ()  [unwired: 1 out]
        }
      }
      n227 = local read "refnum out"() -> (w350:refnum<file>)
      n228 = Close File(refnum=w350, error in=w343) -> (error out=w349:errorcluster)  [unwired: 1 out]
      n229 = property on="Запись в файл" class="Bool (strict)"(error in=w349, "Value"=w342) -> (error out=w348:errorcluster)  [unwired: 1 in, 1 out]
      n230 = local write "Связь с блоком"(w342) -> ()
      n231 = flat-sequence {
        tunnel: w348 -> [w353]
        tunnel: [w353] -> w344
        frame #0 {
          n232 = Stop(stop? (T)=TRUE) -> ()
        }
      }
      n233 = call <vilib>:"General Error Handler.vi"("error in (no error)"=w344, "[exception action] (none:0)"=w345) -> ()  [unwired: 2 in, 12 out]
    }
  }
  n234 = call <vilib>:"Application Directory.vi"() -> ("Application Directory"=w31:path)
  n235 = Path To String(path=w31) -> (string=w32:string)
  n236 = local write "счетчик"(u8 0 ("счетчик")) -> ()
  n237 = Concatenate Strings(w32, "\\IP.txt" ("prompt (Open existing file)")) -> (w33:string)
  n238 = String To Path(string=w33) -> (path=w35:path)
  n239 = local write "stop"(FALSE ("Boolean")) -> ()
  n240 = Read from Text File(file (use dialog)=w35) -> (refnum out=w24:refnum<file>, text=w37:string, error out=w3:errorcluster)  [unwired: 3 in, 1 out]
  n241 = property on="Graphs T" class="WFChart (strict)"("YScale.ScaleFit"=u8 2 ("Y Scale.Scale Fit")) -> (error out=w11:errorcluster)  [unwired: 2 in, 1 out]
  n242 = property on="мин." class="Str"("Disabled"=w46) -> (error out=w45:errorcluster)  [unwired: 2 in, 1 out]
  n243 = property on="К стр." class="Clust (strict)"("DisabledEnum"=w2) -> ()  [unwired: 2 in, 2 out]
  n244 = property on="К спаи" class="Clust (strict)"("DisabledEnum"=w2) -> ()  [unwired: 2 in, 2 out]
  n245 = Match Pattern(string=w37, regular expression="*") -> (after substring=w16:string)  [unwired: 1 in, 3 out]
  n246 = Match Pattern(string=w37, regular expression="%") -> (after substring=w30:string)  [unwired: 1 in, 3 out]
  n247 = invoke on="Graphs T" class="WFChart (strict)" method="Reinit To Default"(error in=w11) -> (error out=w7:errorcluster)  [unwired: 2 in, 2 out]
  n248 = property on="часы" class="Str"(error in=w45, "Disabled"=w46) -> (error out=w44:errorcluster)  [unwired: 1 in, 1 out]
  n249 = property on="К сол." class="Clust (strict)"("DisabledEnum"=w2) -> ()  [unwired: 2 in, 2 out]
  n250 = property on="К пер." class="Clust (strict)"("DisabledEnum"=w2) -> ()  [unwired: 2 in, 2 out]
  n251 = Match Pattern(string=w16, regular expression="--" ("string")) -> (before substring=w15:string)  [unwired: 1 in, 3 out]
  n252 = invoke on="Добавить время" class="Ring (strict)" method="Reinit To Default"(error in=w44) -> (error out=w42:errorcluster)  [unwired: 2 in, 2 out]
  n253 = Match Pattern(string=w30, regular expression="-" ("string")) -> (before substring=w29:string)  [unwired: 1 in, 3 out]
  n254 = Scan From String(format string="%d", input string=w15, default 1=u16 0 ("default value 1")) -> (error out=w14:errorcluster, output 1=w28:u16)  [unwired: 2 in, 2 out]
  n255 = property on="Graphs T" class="WFChart (strict)"(error in=w7, "Value"=dynamicdata [{"t0"=timestamp(3465273261.7246556 s since 1904-01-01), "dt"=1.0, "Y"=[0.1931097262457384]}, {"t0"=timestamp(3465273261.7246556 s since 1904-01-01), "dt"=1.0, "Y"=[0.3594116459482981]}, {"t0"=timestamp(3465273261.7246556 s since 1904-01-01), "dt"=1.0, "Y"=[0.8898205452798131]}, {"t0"=timestamp(3465273261.7246556 s since 1904-01-01), "dt"=1.0, "Y"=[0.747699236883661]}] ("Graphs")) -> (error out=w8:errorcluster)  [unwired: 1 in, 1 out]
  n256 = Merge Errors(w14, w3) -> (w27:errorcluster)
  n257 = property on="save_coeff." class="Bool (strict)"("DisabledEnum"=w2) -> ()  [unwired: 2 in, 2 out]
  n258 = invoke on="File header exist?" class="Bool (strict)" method="Reinit To Default"(error in=w42) -> (error out=w43:errorcluster)  [unwired: 2 in, 2 out]
  n259 = case shown="No Error" w27 {
    selector: w27 -> [w357 w360]
    tunnel: w29 -> [w359 _]
    tunnel: w28 -> [w358 _]
    tunnel: [w359 "?"] -> w26
    tunnel: [w358 u16 0 ("default value 1")] -> w25
    tunnel: w24 -> [w356 w361]
    tunnel: [w356 w361] -> w23
    tunnel: [w357 w360] -> w22
    frame No Error {
    }
    frame Error {
    }
  }
  n260 = property on="load_coeff." class="Bool (strict)"("DisabledEnum"=w2) -> (error out=w38:errorcluster)  [unwired: 2 in, 1 out]
  n261 = property on="Graphs T" class="WFChart (strict)"(error in=w8, "History Data"=dynamicdata[] []) -> (error out=w5:errorcluster)  [unwired: 1 in, 1 out]
  n262 = property on="Расположение файла" class="Path"(error in=w43, "Disabled"=u8 2) -> ()  [unwired: 1 in, 2 out]
  n263 = property on="load_coeff." class="Bool (strict)"(error in=w38, "Val(Sgnl)"=TRUE ("Value (Signaling)")) -> ()  [unwired: 1 in, 2 out]
  n264 = property on="Graphs T" class="WFChart (strict)"(error in=w5, "XScale.ScaleFit"=u8 0 ("Y Scale.Scale Fit")) -> ()  [unwired: 1 in, 2 out]
  n265 = local write "IP"(w26) -> ()
  n266 = local write "Порт"(w25) -> ()
  n267 = Close File(refnum=w23, error in=w22) -> (error out=w21:errorcluster)  [unwired: 1 out]
  n268 = property on="Graphs T" class="WFChart (strict)" props=["XScale", "Minimum"]() -> ()  [unwired: 2 in, 3 out]
  n269 = property on="Graphs T" class="WFChart (strict)" props=["XScale", "Maximum"]() -> ()  [unwired: 2 in, 3 out]
  n270 = call <vilib>:"General Error Handler.vi"("type of dialog (OK msg:1)"=w12, "error in (no error)"=w21) -> ()  [unwired: 1 in, 13 out]
  "File header exist?" <- FALSE ("flag1")
